vi "SnoPowerCompressor.vi"() -> (0 "CompressorValue":bool)   [LabVIEW 2013]
uses:
  <vilib>/Rock Robotics/WPI/Relay/WPI_RelayValue.ctl
  Robot Global Data.vi
panel:
  out "Robot Driving":bool
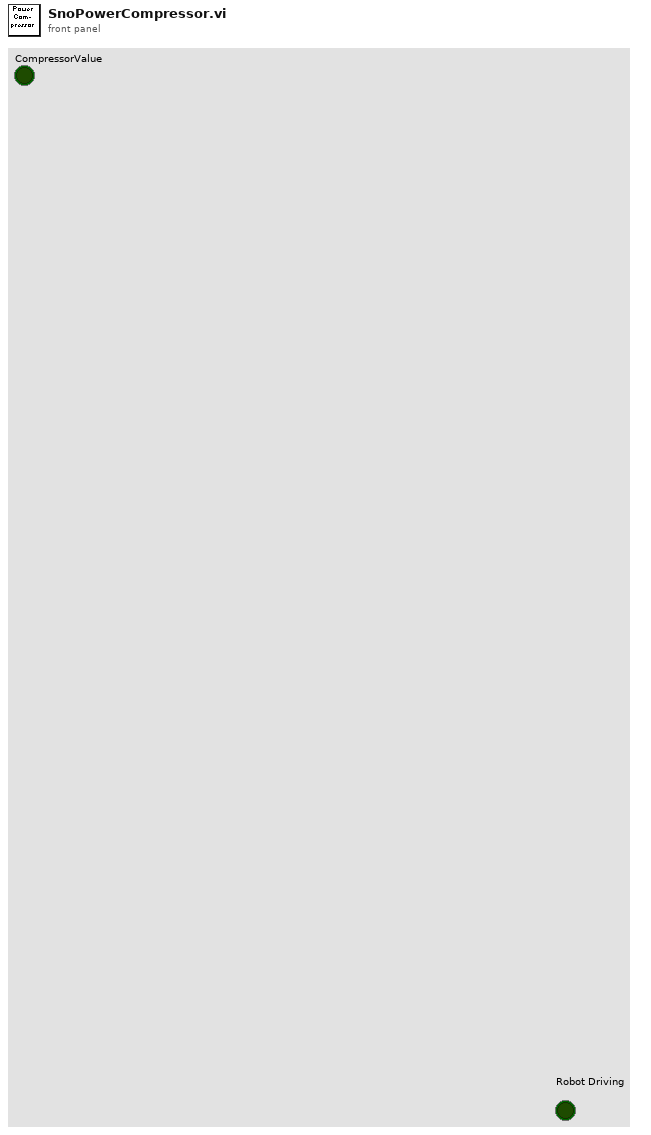
[diagram p1: front panel]
types:
  T1 = typedef "WPI_RelayValue.ctl" = enum16{"Off", "On", "Forward", "Reverse"}
  T2 = typedef "WPI_DigitalInputDevRef.ctl" = cluster{"DevStatus":errorcluster, "DIO Channel":T3, "Digital Module":T4}
  T3 = typedef "FPGA_DIOChannel.ctl" = enum8{"DIO 1", "DIO 2", "DIO 3", "DIO 4", "DIO 5", "DIO 6", "DIO 7", "DIO 8", "DIO 9", "DIO 10", "DIO 11", "DIO 12", "DIO 13", "DIO 14", "Invalid"}
  T4 = typedef "FPGA_TypedefDigitalModule.ctl" = enum16{"Digital Module 1", "Digital Module 2"}
  T5 = typedef "WPI_RelayDevRef.ctl" = cluster{"DevStatus":errorcluster, "Relay Channel":T6, "Digital Module":T4, "Relay Direction":T7}
  T6 = typedef "FPGA_DIORelayChannel.ctl" = enum8{"Relay 1", "Relay 2", "Relay 3", "Relay 4", "Relay 5", "Relay 6", "Relay 7", "Relay 8", "Invalid"}
  T7 = typedef "WPI_RelayDirection.ctl" = enum16{"Both directions", "Forward only", "Reverse only"}
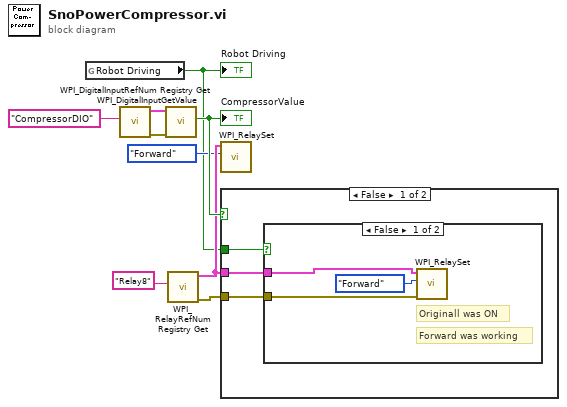
[diagram p0: block diagram]
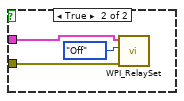
[diagram p2: hidden frame]
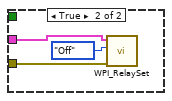
[diagram p3: hidden frame]
diagram:
  n1 = global read "Robot Global Data.vi" "Robot Driving"() -> (w1:bool)
  "Robot Driving" <- w1
  n2 = call <vilib>:"WPI_DigitalInputRefNum Registry Get.vi"("refnum name"="CompressorDIO") -> ("error out"=w6:errorcluster, "DigitalInputDevRef"=w5:T2)  [unwired: 9 in]
  n3 = call <vilib>:"WPI_DigitalInputGetValue.vi"("error in (no error)"=w6, "DigitalInputDevRef"=w5) -> ("Value"=w9:bool)  [unwired: 7 in, 2 out]
  "CompressorValue" <- w9
  n4 = call <vilib>:"WPI_RelayRefNum Registry Get.vi"("refnum name"="Relay8") -> ("error out"=w8:errorcluster, "RelayDevRef"=w3:T5)  [unwired: 9 in]
  n5 = call <vilib>:"WPI_RelaySet.vi"("RelayValue"=WPI_RelayValue."Forward", "RelayDevRef"=w3) -> ()  [unwired: 8 in, 2 out]
  n6 = case shown="False" w9 {
    tunnel: w3 -> [w11 w20]
    tunnel: w8 -> [w10 w19]
    tunnel: w1 -> [w12 _]
    frame False {
      n7 = case shown="False" w12 {
        tunnel: w11 -> [w14 w17]
        tunnel: w10 -> [w13 w16]
        frame False {
          # "Forward was working"
          # "Originall was ON"
          n8 = call <vilib>:"WPI_RelaySet.vi"("error in (no error)"=w13, "RelayValue"=WPI_RelayValue."Forward", "RelayDevRef"=w14) -> ()  [unwired: 7 in, 2 out]
        }
        frame True {
          n9 = call <vilib>:"WPI_RelaySet.vi"("error in (no error)"=w16, "RelayValue"=WPI_RelayValue."Off", "RelayDevRef"=w17) -> ()  [unwired: 7 in, 2 out]
        }
      }
    }
    frame True {
      n10 = call <vilib>:"WPI_RelaySet.vi"("error in (no error)"=w19, "RelayValue"=WPI_RelayValue."Off", "RelayDevRef"=w20) -> ()  [unwired: 7 in, 2 out]
    }
  }
